vi "Update directories.vi"(2 "Source directory":path=path "C:/Documents and Settings/mw24/My Documents/LabVIEW Data/enviroapps") -> (0 "Current file":string)   [LabVIEW 2010]
panel:
  out "Current destination":string
  out "trying to delete file":bool
  in  "distination directories":path[](array[path])=[path "\\\\Enviro\\enviro/Software/RunTime7", path "\\\\ceeserver.cee.cornell.edu\\mw24/Software/Runtime7"]
  in  "stop":bool
  out "file names":string[](array[string])
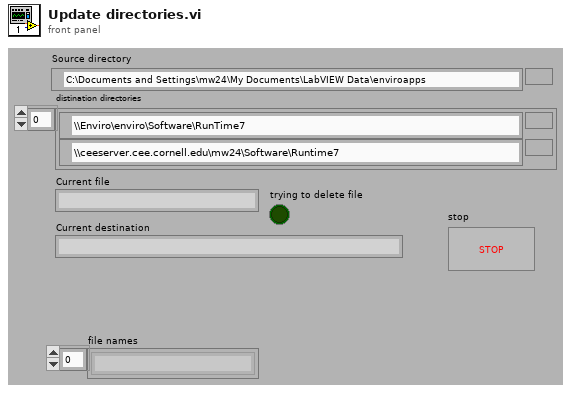
[diagram p1: front panel]
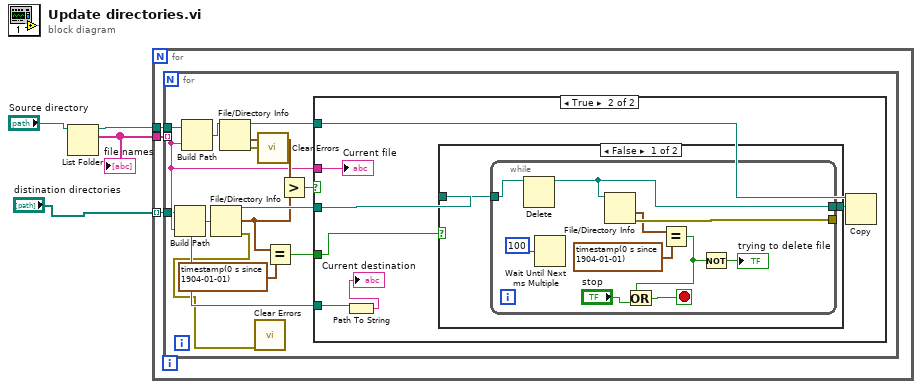
[diagram p0: block diagram]
diagram:
  n1 = List Folder(path="Source directory") -> (path out=w2:path, filenames=w3:string[])  [unwired: 3 in, 2 out]
  "file names" <- w3
  n2 = for {
    tunnel: w3 -> [w7]
    tunnel: w2 -> [w6]
    tunnel: "distination directories" -> [w5] mode=indexing
    n3 = for {
      tunnel: w7 -> [w14] mode=indexing
      tunnel: w6 -> [w21]
      tunnel: w5 -> [w12]
      n4 = Build Path(base path=w12, name or relative path=w14) -> (appended path=w19:path)
      n5 = Build Path(base path=w21, name or relative path=w14) -> (appended path=w20:path)
      n6 = File/Directory Info(path=w19) -> (path out=w17:path, last mod=w10:timestamp, error out=w8:errorcluster)  [unwired: 1 in, 4 out]
      n7 = File/Directory Info(path=w20) -> (path out=w15:path, last mod=w16:timestamp, error out=w13:errorcluster)  [unwired: 1 in, 4 out]
      n8 = call <vilib>:"Clear Errors.vi"("error in (no error)"=w8) -> ()  [unwired: 6 in, 1 out]
      n9 = call <vilib>:"Clear Errors.vi"("error in (no error)"=w13) -> ()  [unwired: 6 in, 1 out]
      n10 = Equal?(x=w10, y=timestamp(0 s since 1904-01-01) ("last mod")) -> (x = y?=w9:bool)
      n11 = Greater?(x=w16, y=w10) -> (0:w18:bool)
      n12 = case shown="True" w18 {
        tunnel: w15 -> [_ w26]
        tunnel: w17 -> [_ w25]
        tunnel: w14 -> [_ w28]
        tunnel: w12 -> [_ w23]
        tunnel: w9 -> [_ w24]
        frame False {
        }
        frame True {
          n13 = Path To String(path=w23) -> (string=→"Current destination":string)
          n14 = case shown="False" w24 {
            tunnel: w25 -> [w30 w41]
            tunnel: [w29 w41] -> w27
            frame False {
              n15 = while {
                tunnel: w30 -> [w40]
                tunnel: [w36] -> w29
                tunnel: [w35] -> _
                stop <- w38 stop-if-true
                n16 = Delete(path (use dialog)=w40) -> (deleted path=w36:path)  [unwired: 4 in, 2 out]
                n17 = Wait Until Next ms Multiple(millisecond multiple=u32 100) -> ()  [unwired: 1 out]
                n18 = File/Directory Info(path=w36) -> (last mod=w33:timestamp, error out=w35:errorcluster)  [unwired: 1 in, 5 out]
                n19 = Equal?(x=w33, y=timestamp(0 s since 1904-01-01) ("last mod")) -> (x = y?=w32:bool)
                n20 = Or(x=w32, y="stop") -> (x .or. y?=w38:bool)
                n21 = Not(x=w32) -> (.not. x?=→"trying to delete file":bool)
              }
            }
            frame True {
              # "File doesn't exist"
            }
          }
          n22 = Copy(10:w27, 11:w26) -> ()  [unwired: 3 in, 3 out]
          "Current file" <- w28
        }
      }
    }
  }
